vi "Keithley2100.measure AC current.vi"(0 "i ref in":refnum<vi>, 1 "Custom Range (100mV)":dbl=0.1 min=0.1 max=1000.0 format="%#.6e", 2 "Digital Filter (0: Off)":u16(ring) items=["Off", "Moving Filter", "Repeating Filter"], 3 "Digital Filter Readings (10)":i32=10, 5 "error in (no error)":errorcluster, 9 "Auto Range":bool) -> (14 "i refout":refnum<vi>, 16 "Measurement":dbl format="%#_6e", 19 "error out":errorcluster)   [LabVIEW 2014, in "Keithley2100.lvlib"]
doc: "This VI is used to get the USB port of the USBSwitchBox from the database.\n\nLicense Agreement for this software:\n\nCopyright (C)\nGesellschaft für Schwerionenforschung, GSI\nPlanckstr. 1\n64291 Darmstadt\nGermany\n\nContact: D.Beck@gsi.de \n\nThis program is free software; you can redistribute it and/or modify it under the terms of the \nGNU General Public License as published by the Free Software Foundation; either version 2 of \nthe license, or (at your option) any later version.\n\nThis program is distributed in the hope that it will be useful, but WITHOUT ANY WARRANTY; \nwithout even the implied warranty of MERCHANTABILITY or FITNESS FOR A PARTICULAR PURPOSE. See the GNU General License for more details (http://www.gnu.org).\n\nGesellschaft für Schwerionenforschung, GSI\nPlanckstr. 1, 64291 Darmstadt, Germany\nFor all questions and ideas contact: M.Richter@gsi.de, H.Brand@gsi.de or D.Beck@gsi.de.\nLast update: 16-JUN-2004"
uses:
  Keithley2100.lvlib
  instr.lib/Keithley-2100-Series/Keithley 2100 Series.lvlib
  CSlibraries-extern/DimLVEvent/LVDimInterface/LVDimInterface.lvlib
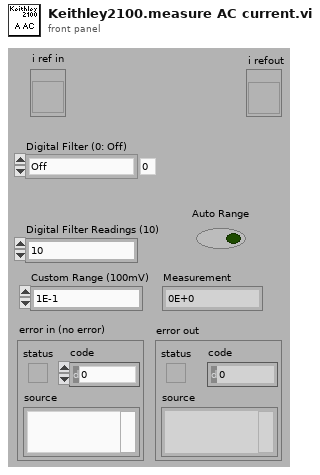
[diagram p1: front panel]
types:
  T1 = typedef "Keithley2100.lvlib/Keithley2100.i attribute.ctl" = cluster{"Custom Range":dbl, "Threshold Range":dbl, "VISA resource name":refnum<visa-resource-name>, "Auto Range":bool, "Digital Filter Readings":i32, "Digital Filter":u16, "NPLC":u16, "Display on":u16, "Resolution":u16, "Beaper enabled":bool, "MeasurementID":i32}
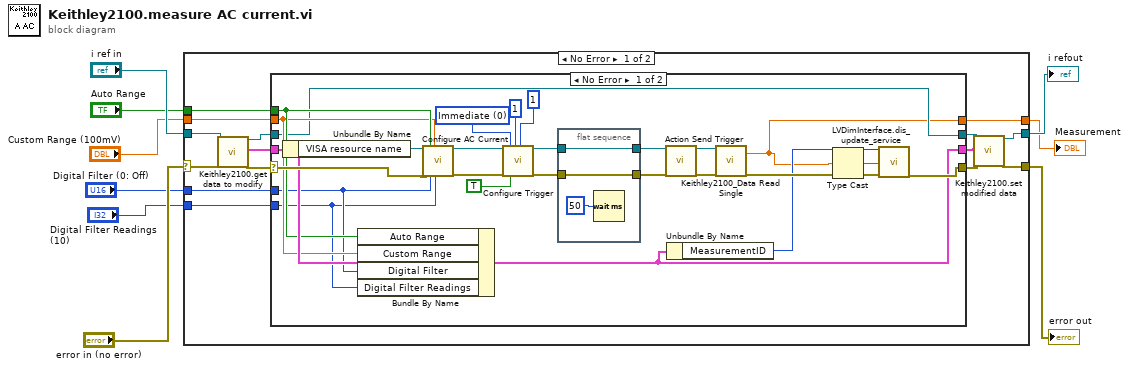
[diagram p0: block diagram]
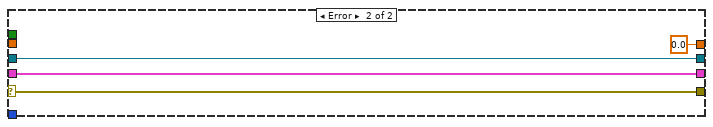
[diagram p2: hidden frame]
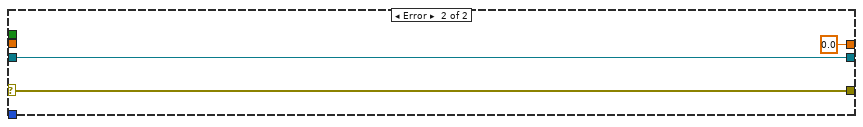
[diagram p3: hidden frame]
diagram:
  n1 = case shown="No Error" "error in (no error)" {
    selector: "error in (no error)" -> [w23 w60]
    tunnel: [w18 w60] -> w7
    tunnel: "i ref in" -> [w24 w59]
    tunnel: [w19 w59] -> w6
    tunnel: "Auto Range" -> [w14 _]
    tunnel: "Custom Range (100mV)" -> [w13 _]
    tunnel: "Digital Filter (0: Off)" -> [w12 _]
    tunnel: "Digital Filter Readings (10)" -> [w11 _]
    tunnel: [w10 0.0 ("Measurement")] -> w1
    frame No Error {
      n2 = call "Keithley2100.get data to modify.vi"("i ref in"=w24, "error in (no error)"=w23) -> ("i ref out"=w21:refnum<vi>, "i attribute"=w20:T1, "error out"=w22:errorcluster)  [unwired: 14 in, 1 out]
      n3 = case shown="No Error" w22 {
        selector: w22 -> [w49 w56]
        tunnel: w21 -> [w31 w57]
        tunnel: w20 -> [w48 w55]
        tunnel: [w31 w57] -> w17
        tunnel: [w29 w56] -> w16
        tunnel: [w28 w55] -> w15
        tunnel: w14 -> [w47 _]
        tunnel: w13 -> [w46 _]
        tunnel: w12 -> [w45 _]
        tunnel: w11 -> [w44 _]
        tunnel: [w26 0.0 ("Measurement")] -> w10
        frame No Error {
          w39 = u16 0 items=["Immediate", "Bus", "External"] ("Source (0: Immediate)")
          n4 = Unbundle By Name(w48) -> ("VISA resource name"=w50:refnum<visa-resource-name>)
          n5 = Bundle By Name(cluster=w48, "Auto Range"=w47, "Custom Range"=w46, "Digital Filter"=w45, "Digital Filter Readings"=w44) -> (w28:T1)
          n6 = call "Configure AC Current.vi"("VISA resource name"=w50, "error in (no error)"=w49, "Auto Range? (T: Auto)"=w47, "Digital Filter (0: Off)"=w45, "Custom Range (0 A)"=w46, "Digital Filter Readings (10)"=w44) -> ("VISA resource name out"=w43:refnum<visa-resource-name>, "error out"=w42:errorcluster)  [unwired: 12 in]
          n7 = call "Configure Trigger.vi"("VISA resource name"=w43, "error in (no error)"=w42, "Source (0: Immediate)"=w39, "Auto Delay? (T: Auto)"=TRUE, "Sample Count (1)"=1, "Trigger Count (1)"=1) -> ("VISA resource name out"=w37:refnum<visa-resource-name>, "error out"=w36:errorcluster)  [unwired: 12 in]
          n8 = flat-sequence {
            tunnel: [w52] -> w35
            tunnel: w37 -> [w52]
            tunnel: [w51] -> w34
            tunnel: w36 -> [w51]
            frame #0 {
              n9 = Wait (ms)(milliseconds to wait=u32 50) -> ()  [unwired: 1 out]
            }
          }
          n10 = call "Action Send Trigger.vi"("VISA resource name"=w35, "error in (no error)"=w34) -> ("VISA resource name out"=w33:refnum<visa-resource-name>, "error out"=w32:errorcluster)  [unwired: 16 in]
          n11 = Unbundle By Name(w28) -> ("MeasurementID"=w27:i32)
          n12 = call "Keithley2100_Data Read Single.vi"("VISA resource name"=w33, "error in (no error)"=w32) -> ("Measurement"=w26:dbl, "error out"=w30:errorcluster)  [unwired: 15 in, 1 out]
          n13 = Type Cast(x=w26) -> (*(type *) &x=w25:string)  [unwired: 1 in]
          n14 = call "LVDimInterface.dis_update_service.vi"("my_serviceID"=w27, "data"=w25, "error in (no error)"=w30) -> ("error out"=w29:errorcluster)  [unwired: 14 in, 2 out]
        }
        frame Error {
        }
      }
      n15 = call "Keithley2100.set modified data.vi"("i ref in"=w17, "i attribute"=w15, "error in (no error)"=w16) -> ("i ref out"=w19:refnum<vi>, "error out"=w18:errorcluster)  [unwired: 15 in]
    }
    frame Error {
    }
  }
  "error out" <- w7
  "i refout" <- w6
  "Measurement" <- w1
